vi "Create.vi"(8 "error in (no error)":errorcluster, 10 "Update Bind":refnum<user-event>) -> (0 "error out":errorcluster, 3 "ControlBindingPanel out":refnum<class "ControlBindingPanel.lvclass">)   [LabVIEW 2020, in "VolatusGUIEditor.lvlib" / "ControlBindingPanel.lvclass"]
uses:
  ControlBindingPanel.lvclass
  ControlBindingPanel.lvclass/ControlBindingPanel.ctl
  Control Bind Data.ctl
  VolatusGUIControls/VolatusGUIControls.lvlib
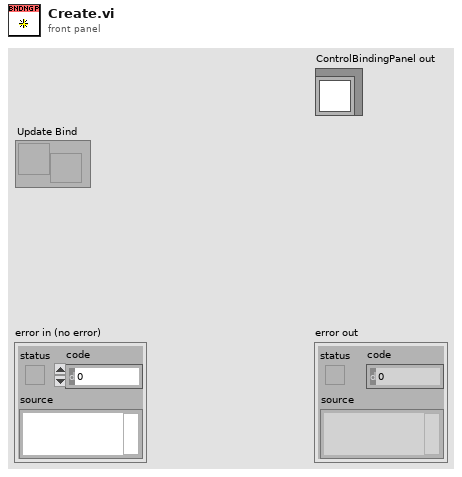
[diagram p1: front panel]
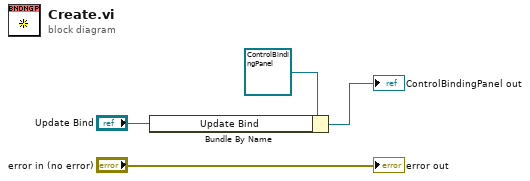
[diagram p0: block diagram]
diagram:
  n1 = Bundle By Name(cluster=refnum<class "ControlBindingPanel.lvclass"> refnum ("ControlBindingPanel in"), "Update Bind"="Update Bind") -> (→"ControlBindingPanel out":refnum<class "ControlBindingPanel.lvclass">)
  "error out" <- "error in (no error)"
